vi "OBD_init.vi"(8 "error in":errorcluster, 10 "COM port":refnum<visa-resource-name>="COM2") -> (0 "error out":errorcluster, 2 "OBD enabled":bool=TRUE)   [LabVIEW 2020]
doc: "Initialize OBD communication"
uses:
  <vilib>/Instr/_visa.llb/VISA Configure Serial Port (Instr).vi
  terminal_test.vi
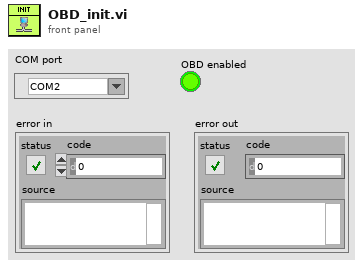
[diagram p1: front panel]
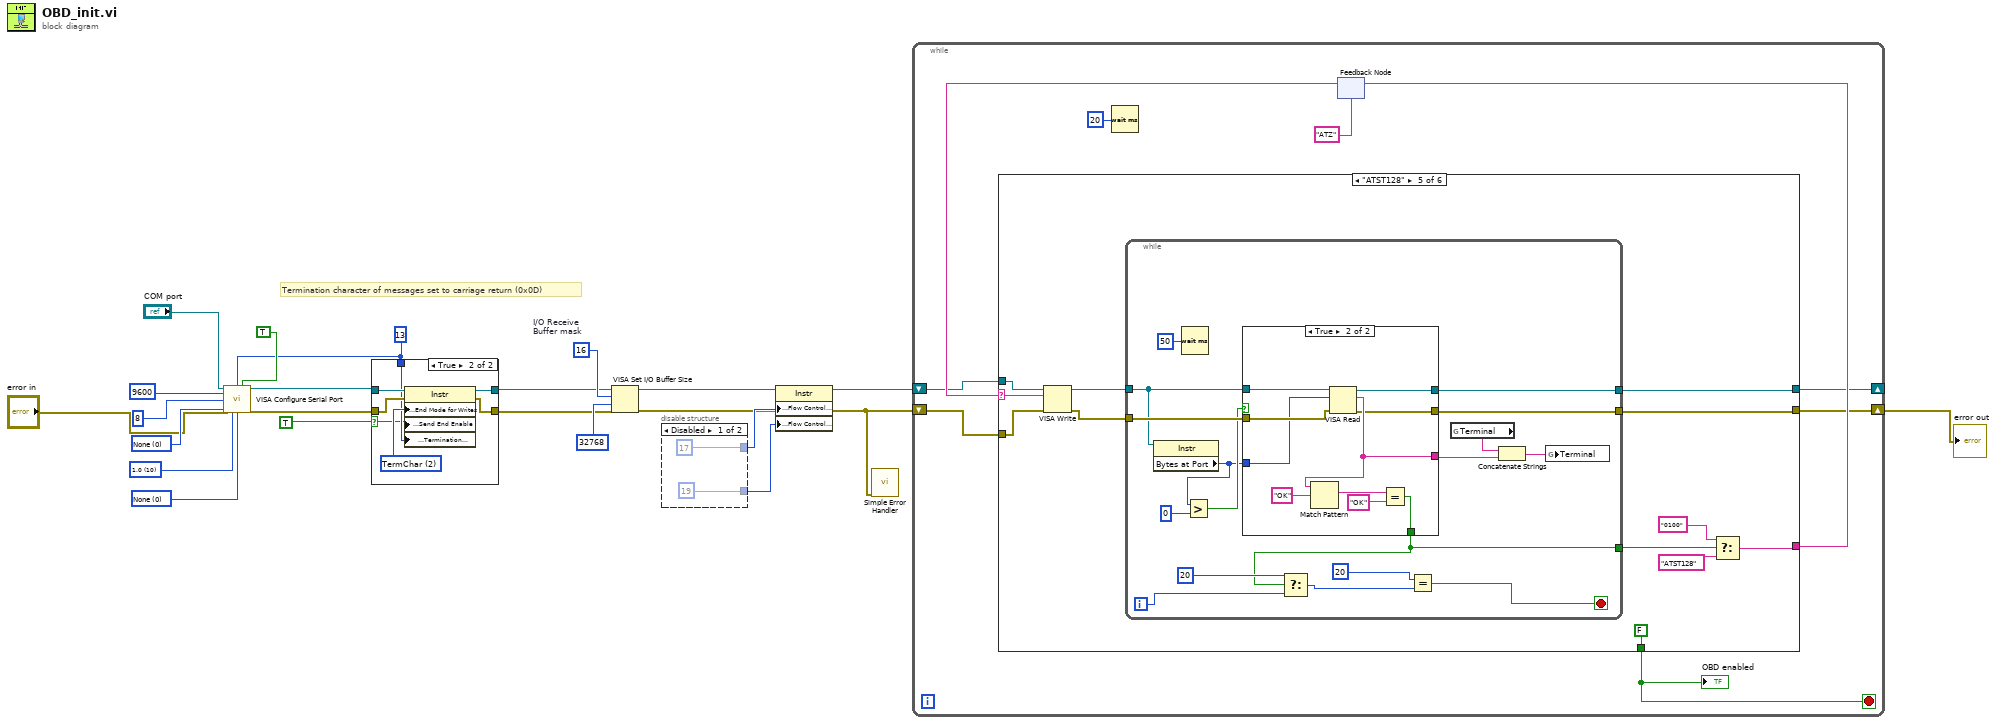
[diagram p0: block diagram]
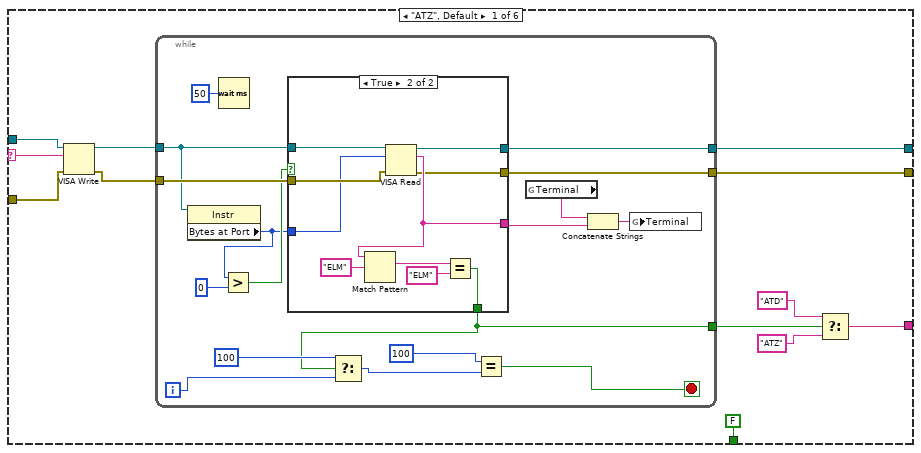
[diagram p4: hidden frame]
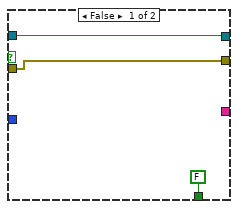
[diagram p5: hidden frame]
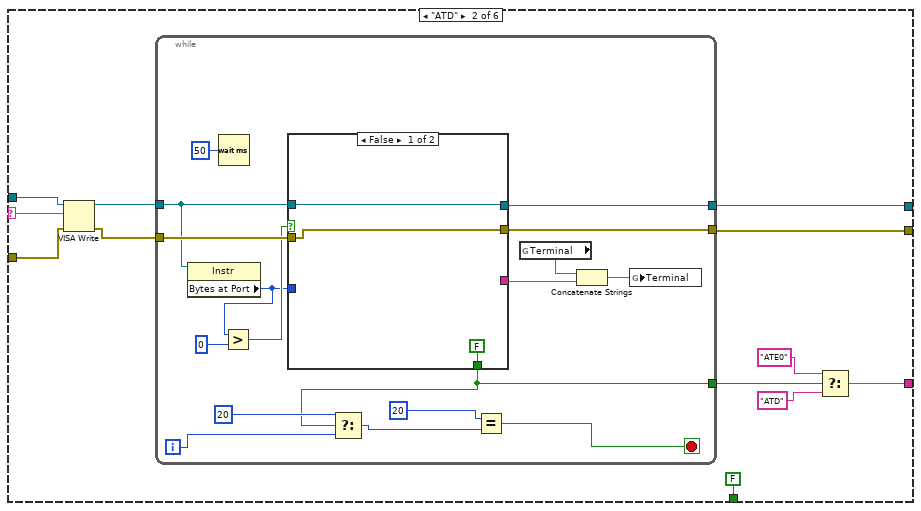
[diagram p6: hidden frame]
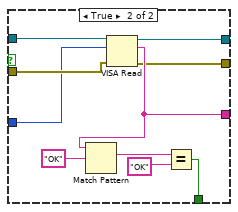
[diagram p7: hidden frame]
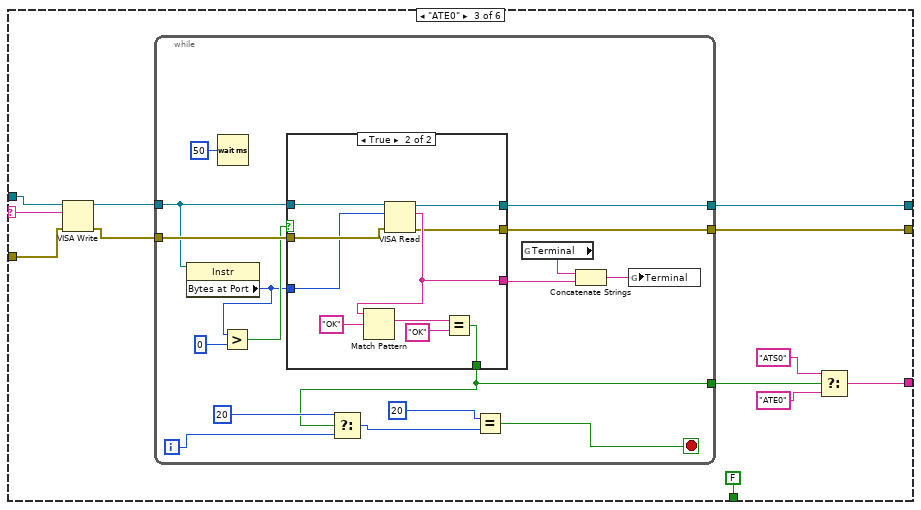
[diagram p8: hidden frame]
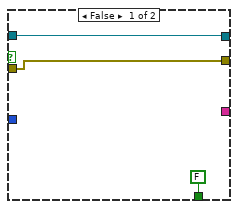
[diagram p9: hidden frame]
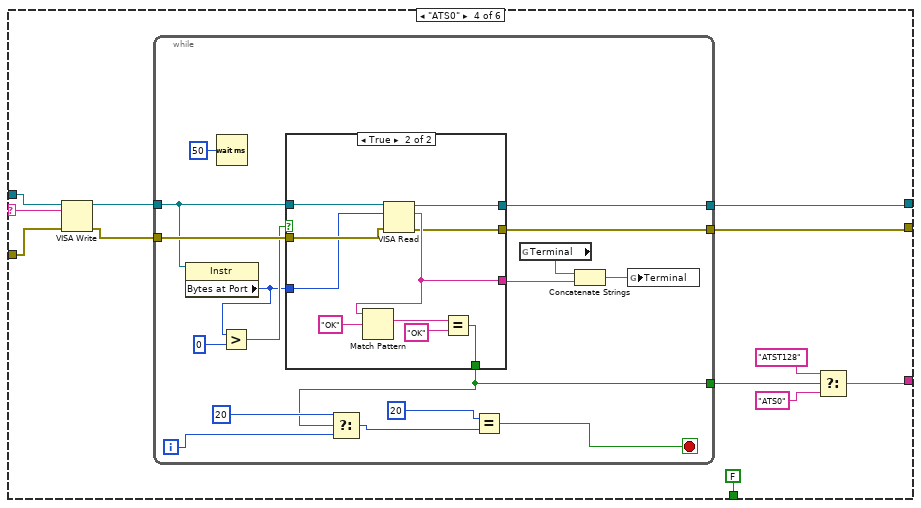
[diagram p10: hidden frame]
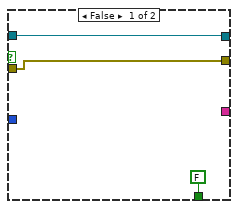
[diagram p11: hidden frame]
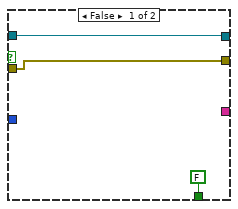
[diagram p12: hidden frame]
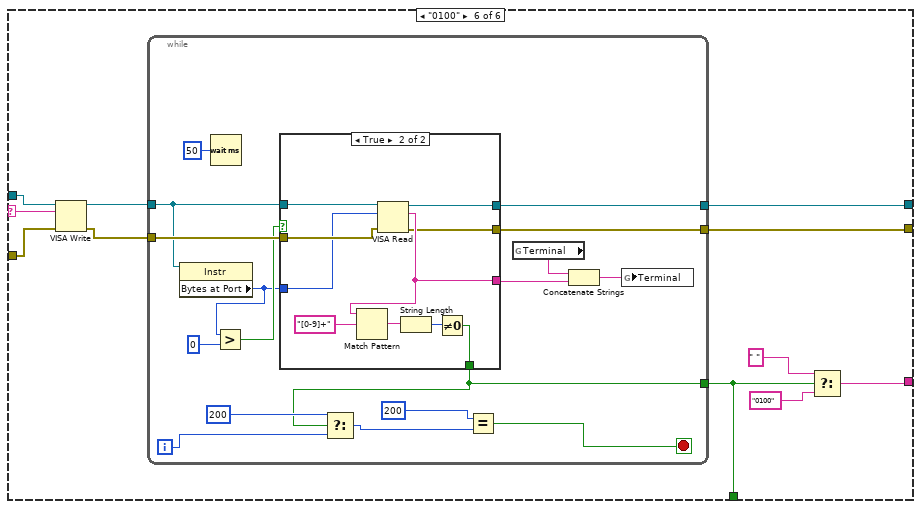
[diagram p13: hidden frame]
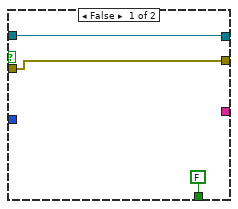
[diagram p14: hidden frame]
diagram:
  w15 = u16 0 items=["None"=0, "XON/XOFF"=1, "RTS/CTS"=2, "DTR/DSR"=4] ("flow control")
  w19 = u16 10 items=["1.0"=10, "1.5"=15, "2.0"=20] ("stop bits")
  w9 = u8 13 ("termination char\n(0xA = '\\n' = LF)")
  w20 = u16 0 items=["None", "Odd", "Even", "Mark", "Space"] ("parity")
  w10 = u16 16  # I/O Receive Buffer mask
  # "Termination character of messages set to carriage return (0x0D)"
  n1 = call-poly "VISA Configure Serial Port"("VISA resource name"="COM port", "termination char\n(0xA = '\\n' = LF)"=w9, "Enable Termination\nChar (T)"=TRUE ("End read on termination character?"), "baud rate (9600)"=u32 9600 ("baud rate"), "data bits (8)"=u16 8 ("data bits"), "parity (0:none)"=w20, "error in (no error)"="error in", "stop bits (10: 1 bit)"=w19, "flow control (0:none)"=w15) -> ("VISA resource name out"=w11:refnum<visa-resource-name>, "error out"=w13:errorcluster)  [unwired: 1 in, 4 out]
  n2 = case shown="True" TRUE ("End write with termination character?") {
    selector: TRUE ("End write with termination character?") -> [_ w25]
    tunnel: w11 -> [w23 w31]
    tunnel: w13 -> [w24 w30]
    tunnel: [w23 w29] -> w5
    tunnel: [w24 w28] -> w12
    tunnel: w9 -> [_ w26]
    frame False {
    }
    frame True {
      w27 = u16 2 items=["None", "LastBit", "TermChar", "Break"] ("Serial Settings:Serial End Mode for Writes")
      n3 = property class="Instr"(reference=w31, error in=w30, "Serial Settings:End Mode for Writes"=w27, "Message Based Settings:Send End Enable"=w25, "Message Based Settings:Termination Character"=w26) -> (reference out=w29:refnum<visa-resource-name>, error out=w28:errorcluster)
    }
  }
  n4 = VISA Set I/O Buffer Size(VISA resource name=w5, mask (16)=w10, size (4096)=u32 32768 ("Input\nbuffer size"), error in (no error)=w12) -> (VISA resource name out=w6:refnum<visa-resource-name>, error out=w1:errorcluster)
  n5 = disable-structure shown="Disabled" {
    disable-tunnel: [u8 17 ("XON Character") _] -> w8
    disable-tunnel: [u8 19 ("XOFF Character") _] -> w7
    frame Disabled {
    }
    frame Enabled {
    }
  }
  n6 = property class="Instr"(reference=w6, "Serial Settings:Flow Control XON Character"=w8, "Serial Settings:Flow Control XOFF Character"=w7) -> (reference out=w3:refnum<visa-resource-name>)  [unwired: 1 in, 1 out]
  n7 = call <vilib>:"Simple Error Handler.vi"("error in (no error)"=w1) -> ()  [unwired: 1 in, 8 out]
  n8 = while {
    shift-right: [w37] -> _
    shift-left: w3 -> [w39]
    shift-right: [w36] -> w22
    shift-left: w1 -> [w38]
    stop <- w35 stop-if-true
    n9 = Wait (ms)(milliseconds to wait=u32 20) -> ()  [unwired: 1 out]
    n10 = feedback #1("ATZ") -> (w41:string)
    n11 = case shown="\"ATST128\"" w41 {
      selector: w41 -> [w54 w89 w130 w173 w212 w258]
      tunnel: [w48 w88 w131 w170 w217 w259] -> w40
      tunnel: w39 -> [w47 w91 w129 w175 w214 w257]
      tunnel: w38 -> [w46 w90 w128 w174 w213 w256]
      tunnel: [w45 w87 w133 w172 w215 w255] -> w37
      tunnel: [w44 w86 w132 w171 w216 w254] -> w36
      tunnel: [FALSE FALSE FALSE FALSE FALSE w253] -> w35
      frame "ATZ", Default {
        n12 = VISA Write(VISA resource name=w47, write buffer=w54, error in (no error)=w46) -> (VISA resource name out=w53:refnum<visa-resource-name>, error out=w52:errorcluster)  [unwired: 1 out]
        n13 = while {
          tunnel: w53 -> [w67]
          tunnel: w52 -> [w71]
          tunnel: [w60] -> w51
          tunnel: [w58] -> w45
          tunnel: [w57] -> w44
          i -> [w64]
          stop <- w63 stop-if-true
          n14 = property class="Instr"(reference=w67) -> ("Bytes at Port"=w68:u32)  [unwired: 1 in, 2 out]
          n15 = Wait (ms)(milliseconds to wait=u32 50) -> ()  [unwired: 1 out]
          n16 = Greater?(x=w68, y=u32 0) -> (0:w69:bool)
          n17 = case shown="True" w69 {
            tunnel: w67 -> [w73 w84]
            tunnel: w71 -> [w72 w83]
            tunnel: w68 -> [_ w82]
            tunnel: [FALSE w78] -> w60
            tunnel: [_ w77] -> w59
            tunnel: [w73 w76] -> w58
            tunnel: [w72 w75] -> w57
            frame False {
            }
            frame True {
              n18 = VISA Read(VISA resource name=w84, byte count=w82, error in (no error)=w83) -> (VISA resource name out=w76:refnum<visa-resource-name>, read buffer=w77:string, error out=w75:errorcluster)  [unwired: 1 out]
              n19 = Match Pattern(string=w77, regular expression="ELM") -> (match substring=w79:string)  [unwired: 1 in, 3 out]
              n20 = Equal?(x=w79, y="ELM") -> (x = y?=w78:bool)
            }
          }
          n21 = Select(t=100, s=w60, f=w64) -> (s? t:f=w62:i32)
          n22 = Equal?(x=100, y=w62) -> (x = y?=w63:bool)
          n23 = global read "terminal_test.vi" "Terminal"() -> (w55:string)
          n24 = Concatenate Strings(w55, w59) -> (w56:string)
          n25 = global write "terminal_test.vi" "Terminal"(w56) -> ()
        }
        n26 = Select(t="ATD", s=w51, f="ATZ") -> (s? t:f=w48:string)
      }
      frame "ATD" {
        n27 = VISA Write(VISA resource name=w91, write buffer=w89, error in (no error)=w90) -> (VISA resource name out=w94:refnum<visa-resource-name>, error out=w95:errorcluster)  [unwired: 1 out]
        n28 = while {
          tunnel: w94 -> [w109]
          tunnel: w95 -> [w113]
          tunnel: [w102] -> w96
          tunnel: [w99] -> w87
          tunnel: [w98] -> w86
          i -> [w106]
          stop <- w105 stop-if-true
          n29 = property class="Instr"(reference=w109) -> ("Bytes at Port"=w110:u32)  [unwired: 1 in, 2 out]
          n30 = Wait (ms)(milliseconds to wait=u32 50) -> ()  [unwired: 1 out]
          n31 = Greater?(x=w110, y=u32 0) -> (0:w111:bool)
          n32 = case shown="False" w111 {
            tunnel: w109 -> [w115 w126]
            tunnel: w113 -> [w114 w125]
            tunnel: w110 -> [_ w124]
            tunnel: [FALSE w120] -> w102
            tunnel: [_ w119] -> w101
            tunnel: [w115 w118] -> w99
            tunnel: [w114 w117] -> w98
            frame False {
            }
            frame True {
              n33 = VISA Read(VISA resource name=w126, byte count=w124, error in (no error)=w125) -> (VISA resource name out=w118:refnum<visa-resource-name>, read buffer=w119:string, error out=w117:errorcluster)  [unwired: 1 out]
              n34 = Match Pattern(string=w119, regular expression="OK") -> (match substring=w121:string)  [unwired: 1 in, 3 out]
              n35 = Equal?(x=w121, y="OK") -> (x = y?=w120:bool)
            }
          }
          n36 = Select(t=20, s=w102, f=w106) -> (s? t:f=w104:i32)
          n37 = Equal?(x=20, y=w104) -> (x = y?=w105:bool)
          n38 = global read "terminal_test.vi" "Terminal"() -> (w97:string)
          n39 = Concatenate Strings(w97, w101) -> (w100:string)
          n40 = global write "terminal_test.vi" "Terminal"(w100) -> ()
        }
        n41 = Select(t="ATE0", s=w96, f="ATD") -> (s? t:f=w88:string)
      }
      frame "ATE0" {
        n42 = VISA Write(VISA resource name=w129, write buffer=w130, error in (no error)=w128) -> (VISA resource name out=w138:refnum<visa-resource-name>, error out=w137:errorcluster)  [unwired: 1 out]
        n43 = while {
          tunnel: w138 -> [w151]
          tunnel: w137 -> [w155]
          tunnel: [w144] -> w136
          tunnel: [w141] -> w133
          tunnel: [w140] -> w132
          i -> [w148]
          stop <- w147 stop-if-true
          n44 = property class="Instr"(reference=w151) -> ("Bytes at Port"=w152:u32)  [unwired: 1 in, 2 out]
          n45 = Wait (ms)(milliseconds to wait=u32 50) -> ()  [unwired: 1 out]
          n46 = Greater?(x=w152, y=u32 0) -> (0:w153:bool)
          n47 = case shown="True" w153 {
            tunnel: w151 -> [w157 w168]
            tunnel: w155 -> [w156 w167]
            tunnel: w152 -> [_ w166]
            tunnel: [FALSE w162] -> w144
            tunnel: [_ w161] -> w143
            tunnel: [w157 w160] -> w141
            tunnel: [w156 w159] -> w140
            frame False {
            }
            frame True {
              n48 = VISA Read(VISA resource name=w168, byte count=w166, error in (no error)=w167) -> (VISA resource name out=w160:refnum<visa-resource-name>, read buffer=w161:string, error out=w159:errorcluster)  [unwired: 1 out]
              n49 = Match Pattern(string=w161, regular expression="OK") -> (match substring=w163:string)  [unwired: 1 in, 3 out]
              n50 = Equal?(x=w163, y="OK") -> (x = y?=w162:bool)
            }
          }
          n51 = Select(t=20, s=w144, f=w148) -> (s? t:f=w146:i32)
          n52 = Equal?(x=20, y=w146) -> (x = y?=w147:bool)
          n53 = global read "terminal_test.vi" "Terminal"() -> (w139:string)
          n54 = Concatenate Strings(w139, w143) -> (w142:string)
          n55 = global write "terminal_test.vi" "Terminal"(w142) -> ()
        }
        n56 = Select(t="ATS0", s=w136, f="ATE0") -> (s? t:f=w131:string)
      }
      frame "ATS0" {
        n57 = VISA Write(VISA resource name=w175, write buffer=w173, error in (no error)=w174) -> (VISA resource name out=w178:refnum<visa-resource-name>, error out=w179:errorcluster)  [unwired: 1 out]
        n58 = while {
          tunnel: w178 -> [w193]
          tunnel: w179 -> [w197]
          tunnel: [w186] -> w180
          tunnel: [w183] -> w172
          tunnel: [w182] -> w171
          i -> [w190]
          stop <- w189 stop-if-true
          n59 = property class="Instr"(reference=w193) -> ("Bytes at Port"=w194:u32)  [unwired: 1 in, 2 out]
          n60 = Wait (ms)(milliseconds to wait=u32 50) -> ()  [unwired: 1 out]
          n61 = Greater?(x=w194, y=u32 0) -> (0:w195:bool)
          n62 = case shown="True" w195 {
            tunnel: w193 -> [w199 w210]
            tunnel: w197 -> [w198 w209]
            tunnel: w194 -> [_ w208]
            tunnel: [FALSE w204] -> w186
            tunnel: [_ w203] -> w185
            tunnel: [w199 w202] -> w183
            tunnel: [w198 w201] -> w182
            frame False {
            }
            frame True {
              n63 = VISA Read(VISA resource name=w210, byte count=w208, error in (no error)=w209) -> (VISA resource name out=w202:refnum<visa-resource-name>, read buffer=w203:string, error out=w201:errorcluster)  [unwired: 1 out]
              n64 = Match Pattern(string=w203, regular expression="OK") -> (match substring=w205:string)  [unwired: 1 in, 3 out]
              n65 = Equal?(x=w205, y="OK") -> (x = y?=w204:bool)
            }
          }
          n66 = Select(t=20, s=w186, f=w190) -> (s? t:f=w188:i32)
          n67 = Equal?(x=20, y=w188) -> (x = y?=w189:bool)
          n68 = global read "terminal_test.vi" "Terminal"() -> (w181:string)
          n69 = Concatenate Strings(w181, w185) -> (w184:string)
          n70 = global write "terminal_test.vi" "Terminal"(w184) -> ()
        }
        n71 = Select(t="ATST128", s=w180, f="ATS0") -> (s? t:f=w170:string)
      }
      frame "ATST128" {
        n72 = VISA Write(VISA resource name=w214, write buffer=w212, error in (no error)=w213) -> (VISA resource name out=w222:refnum<visa-resource-name>, error out=w221:errorcluster)  [unwired: 1 out]
        n73 = while {
          tunnel: w222 -> [w235]
          tunnel: w221 -> [w239]
          tunnel: [w228] -> w220
          tunnel: [w225] -> w215
          tunnel: [w224] -> w216
          i -> [w232]
          stop <- w231 stop-if-true
          n74 = property class="Instr"(reference=w235) -> ("Bytes at Port"=w236:u32)  [unwired: 1 in, 2 out]
          n75 = Wait (ms)(milliseconds to wait=u32 50) -> ()  [unwired: 1 out]
          n76 = Greater?(x=w236, y=u32 0) -> (0:w237:bool)
          n77 = case shown="True" w237 {
            tunnel: w235 -> [w241 w252]
            tunnel: w239 -> [w240 w251]
            tunnel: w236 -> [_ w250]
            tunnel: [FALSE w246] -> w228
            tunnel: [_ w245] -> w227
            tunnel: [w241 w244] -> w225
            tunnel: [w240 w243] -> w224
            frame False {
            }
            frame True {
              n78 = VISA Read(VISA resource name=w252, byte count=w250, error in (no error)=w251) -> (VISA resource name out=w244:refnum<visa-resource-name>, read buffer=w245:string, error out=w243:errorcluster)  [unwired: 1 out]
              n79 = Match Pattern(string=w245, regular expression="OK") -> (match substring=w247:string)  [unwired: 1 in, 3 out]
              n80 = Equal?(x=w247, y="OK") -> (x = y?=w246:bool)
            }
          }
          n81 = Select(t=20, s=w228, f=w232) -> (s? t:f=w230:i32)
          n82 = Equal?(x=20, y=w230) -> (x = y?=w231:bool)
          n83 = global read "terminal_test.vi" "Terminal"() -> (w223:string)
          n84 = Concatenate Strings(w223, w227) -> (w226:string)
          n85 = global write "terminal_test.vi" "Terminal"(w226) -> ()
        }
        n86 = Select(t="0100", s=w220, f="ATST128") -> (s? t:f=w217:string)
      }
      frame "0100" {
        n87 = VISA Write(VISA resource name=w257, write buffer=w258, error in (no error)=w256) -> (VISA resource name out=w262:refnum<visa-resource-name>, error out=w263:errorcluster)  [unwired: 1 out]
        n88 = while {
          tunnel: w262 -> [w276]
          tunnel: w263 -> [w280]
          tunnel: [w269] -> w253
          tunnel: [w266] -> w255
          tunnel: [w265] -> w254
          i -> [w273]
          stop <- w272 stop-if-true
          n89 = property class="Instr"(reference=w276) -> ("Bytes at Port"=w277:u32)  [unwired: 1 in, 2 out]
          n90 = Wait (ms)(milliseconds to wait=u32 50) -> ()  [unwired: 1 out]
          n91 = Greater?(x=w277, y=u32 0) -> (0:w278:bool)
          n92 = case shown="True" w278 {
            tunnel: w276 -> [w282 w293]
            tunnel: w280 -> [w281 w292]
            tunnel: w277 -> [_ w291]
            tunnel: [FALSE w290] -> w269
            tunnel: [_ w289] -> w268
            tunnel: [w282 w288] -> w266
            tunnel: [w281 w287] -> w265
            frame False {
            }
            frame True {
              n93 = VISA Read(VISA resource name=w293, byte count=w291, error in (no error)=w292) -> (VISA resource name out=w288:refnum<visa-resource-name>, read buffer=w289:string, error out=w287:errorcluster)  [unwired: 1 out]
              n94 = Match Pattern(string=w289, regular expression="[0-9]+") -> (match substring=w284:string)  [unwired: 1 in, 3 out]
              n95 = String Length(string=w284) -> (length=w285:i32)
              n96 = Not Equal To 0?(x=w285) -> (x != 0?=w290:bool)
            }
          }
          n97 = Select(t=200, s=w269, f=w273) -> (s? t:f=w271:i32)
          n98 = Equal?(x=200, y=w271) -> (x = y?=w272:bool)
          n99 = global read "terminal_test.vi" "Terminal"() -> (w264:string)
          n100 = Concatenate Strings(w264, w268) -> (w267:string)
          n101 = global write "terminal_test.vi" "Terminal"(w267) -> ()
        }
        n102 = Select(t=" ", s=w253, f="0100") -> (s? t:f=w259:string)
      }
    }
    "OBD enabled" <- w35
    n103 = feedback-in #1(w40) -> ()
  }
  "error out" <- w22
